vi "AndorAcqSingleImageToTiff.vi"(7 "Total Images":i32, 8 "Image Nr":i32, 9 "Exposure":sgl=50.0 format="%#_g ms", 10 "Image Name":string, 11 "TiffHandle IN":refnum<k24>) -> (0 "Error Array":cluster{i32, string}[](array[cluster]), 2 "Image":T1, 3 "TiffOut":refnum<k24>)   [LabVIEW 2018]
uses:
  C:/Users/johan/Downloads/LabVIEW software/LabVIEW software/IX-81 Software/lib/TIFF/LVTiffWriter/BitMiracle.LibTiff.NET.dll
  TIFF/LVTiffWriter/BitMiracle.LibTiff.NET.dll
  <vilib>/vision/Image Controls.llb/IMAQ Image.ctl
  Andor SDK/AndorSDK.lvlib
  tiff/LVTiffWriter/LVTiffWriter.lvlib
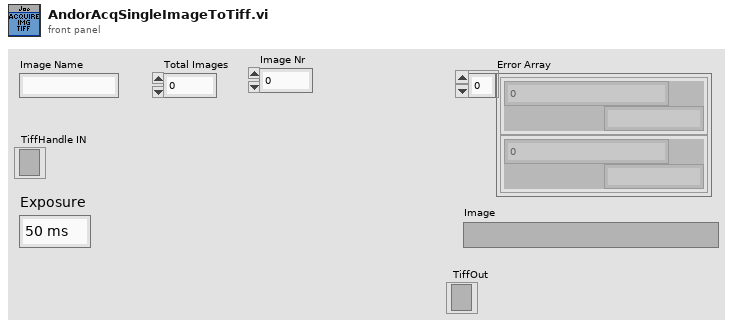
[diagram p1: front panel]
types:
  T1 = typedef "IMAQ Image.ctl" = refnum<image>
  T2 = typedef "Image Type" = u32
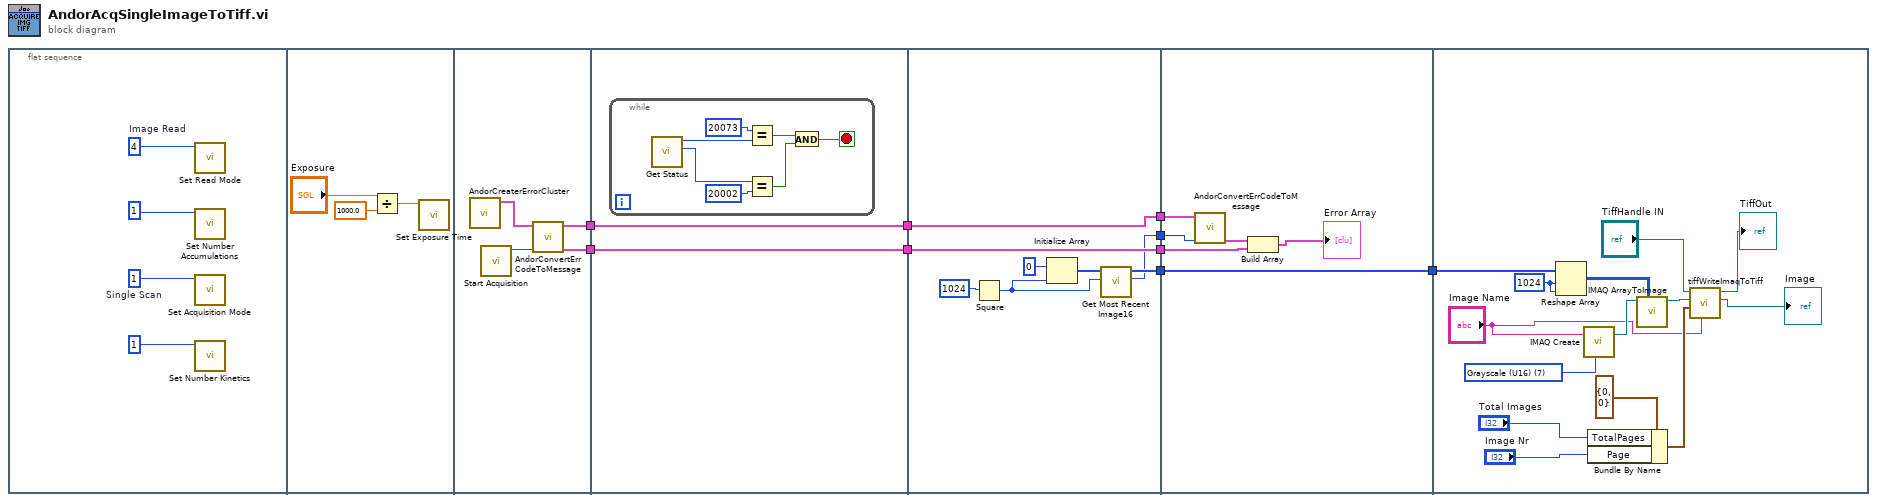
[diagram p0: block diagram]
diagram:
  n1 = flat-sequence {
    tunnel: [w19] -> w9
    tunnel: [w18] -> w8
    tunnel: w9 -> [w21]
    tunnel: w8 -> [w22]
    tunnel: [w22] -> w7
    tunnel: [w21] -> w6
    tunnel: w7 -> [w37]
    tunnel: w6 -> [w36]
    tunnel: [w37] -> w5
    tunnel: [w36] -> w4
    tunnel: [w32] -> w3
    tunnel: [w33] -> w2
    tunnel: w5 -> [w41]
    tunnel: w4 -> [w39]
    tunnel: w3 -> [w40]
    tunnel: w2 -> [w43]
    tunnel: [w43] -> w1
    tunnel: w1 -> [w54]
    frame #0 {
      w10 = 1  # Single Scan
      w11 = 4  # Image Read
      n2 = call "Set Read Mode.vi"("mode"=w11) -> ()  [unwired: 10 in, 1 out]
      n3 = call "Set Number Accumulations.vi"("number"=1) -> ()  [unwired: 10 in, 1 out]
      n4 = call "Set Acquisition Mode.vi"("mode"=w10) -> ()  [unwired: 10 in, 1 out]
      n5 = call "Set Number Kinetics.vi"("number"=1) -> ()  [unwired: 10 in, 1 out]
    }
    frame #1 {
      n6 = Divide(x="Exposure", y=sgl 1000.0) -> (x/y=w15:sgl)
      n7 = call "Set Exposure Time.vi"("time"=w15) -> ()  [unwired: 10 in, 1 out]
    }
    frame #2 {
      n8 = call "AndorCreaterErrorCluster.vi"() -> ("Array"=w17:cluster{i32, string}[])  [unwired: 11 in]
      n9 = call "Start Acquisition.vi"() -> ("function return"=w20:u32)  [unwired: 11 in]
      n10 = call "AndorConvertErrCodeToMessage.vi"("function return"=w20, "Array"=w17) -> ("Element Return"=w18:cluster{i32, string}, "Array out"=w19:cluster{i32, string}[])  [unwired: 8 in]
    }
    frame #3 {
      n11 = while {
        stop <- w23 stop-if-true
        n12 = call "Get Status.vi"() -> ("function return"=w29:u32, "status out"=w26:i32)  [unwired: 10 in]
        n13 = Equal?(x=20073 ("status out"), y=w26) -> (x = y?=w25:bool)
        n14 = Equal?(x=w29, y=20002 ("x")) -> (x = y?=w24:bool)
        n15 = And(x=w25, y=w24) -> (x .and. y?=w23:bool)
      }
    }
    frame #4 {
      n16 = Square(x=1024) -> (x^2=w30:i32)
      n17 = Initialize Array(i16 0 ("element"), w30) -> (w31:i16[])
      n18 = call "Get Most Recent Image16.vi"("size"=w30, "arr"=w31) -> ("function return"=w32:u32, "arr out"=w33:u16[])  [unwired: 7 in, 1 out]
    }
    frame #5 {
      n19 = call "AndorConvertErrCodeToMessage.vi"("function return"=w40, "Array"=w39) -> ("Element Return"=w42:cluster{i32, string})  [unwired: 8 in, 1 out]
      n20 = Build Array(w42, w41) -> (→"Error Array":cluster{i32, string}[])
    }
    frame #6 {
      w56 = T2 7 items=["Grayscale (U8)", "Grayscale (I16)", "Grayscale (SGL)", "Complex (CSG)", "RGB (U32)", "HSL (U32)", "RGB (U64)", "Grayscale (U16)"] ("Image Type")
      w55 = 1024 ("dimension size")
      n21 = Reshape Array(w54, w55, w55) -> (w52:u16[][])
      n22 = call "IMAQ Create"("Image Name"="Image Name", "Image Type"=w56) -> ("New Image"=w57:T1)  [unwired: 3 in, 1 out]
      n23 = Bundle By Name(cluster=cluster{"Page":i32, "TotalPages":i32} {"Page"=0, "TotalPages"=0} ("Multipage"), "TotalPages"="Total Images", "Page"="Image Nr") -> (w47:cluster{"Page":i32, "TotalPages":i32})
      n24 = call "IMAQ ArrayToImage"("Image Pixels (U16)"=w52, "Image"=w57) -> ("Image Out"=w53:T1)  [unwired: 8 in, 1 out]
      n25 = call "tiffWriteImaqToTiff.vi"("ImageDescription"="Image Name", "Multipage"=w47, "ImaqIn"=w53, "TiffIn"="TiffHandle IN") -> ("ImaqOut"=→"Image":T1, "TiffOut"=→"TiffOut":refnum<k24>)  [unwired: 6 in]
    }
  }
